vi "Seven Segment Display.vi"(7 "Seven Seg Type (Common Anode)":enum16{"Common Anode", "Common Cathode"}(ring), 8 "Error In":errorcluster, 9 "Character":string="s", 10 "Channels":u8[](array[numeric]), 11 "LINX Resource":T2) -> (0 "Error Out":errorcluster, 2 "Seven Seg Indicator":T1, 3 "LINX Resource":T2)   [LabVIEW 2020, in "LMH-LINX.lvlib"]
doc: "Write a character to a seven segment display using digital output pins. If a multi character string is pass into 'Character' this vi writest he last character. If the selected character cannot be rendered on a seven segment display all segments will turn off."
uses:
  LMH-LINX.lvlib
  Private/Type Defs/LINX Ref.ctl
  Private/Type Defs/Platform.ctl
  Private/Type Defs/Interface.ctl
  Private/Device/Type Defs/LINX Device Config.ctl
  Private/Device/Type Defs/TCP Config.ctl
  Private/Device/Type Defs/Channels.ctl
  Private/Type Defs/Seven Segment Control.ctl
  Peripherals/Digital/Digital Write N Chans.vi
  Private/Local IO/LinxDigitalWrite.vi
  Utilities/Check Channel.vi
  Private/Utilties/Generate Error.vi
  Private/Device/Device.lvlib
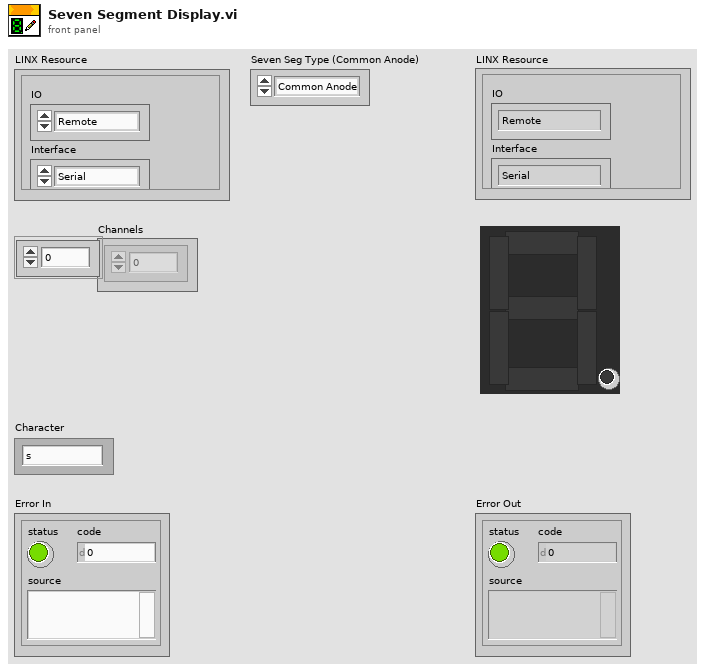
[diagram p1: front panel]
types:
  T1 = typedef "LMH-LINX.lvlib/Seven Segment Control.ctl" = cluster{"Segment 0":bool, "Segment 1":bool, "Segment 2":bool, "Segment 3":bool, "Segment 4":bool, "Segment 5":bool, "Segment 6":bool, "DP":bool}
  T2 = typedef "LMH-LINX.lvlib/LINX Ref.ctl" = cluster{"IO":T3, "Interface":T4, "LINX Device Config":T5}
  T3 = typedef "LMH-LINX.lvlib/Platform.ctl" = enum16{"Remote", "Local"}
  T4 = typedef "LMH-LINX.lvlib/Interface.ctl" = enum16{"Serial", "TCP"}
  T5 = typedef "LMH-LINX.lvlib/Device.lvlib/LINX Device Config.ctl" = cluster{"Interface":T4, "COM Port":refnum<visa-resource-name>, "TCP Configuration":T6, "Device Family":u8, "Device ID":u8, "Device Name":string, "TCP Ref":refnum<k5>, "Channels":T7}
  T6 = typedef "LMH-LINX.lvlib/Device.lvlib/TCP Config.ctl" = cluster{"IP Address":string, "Port":u16}
  T7 = typedef "LMH-LINX.lvlib/Channels.ctl" = cluster{"DI":u8[], "DO":u8[], "AI":u8[], "AO":u8[], "PWM":u8[], "QE":u8[], "UART":u8[], "I2C 2":u8[], "SPI":u8[], "CAN":u8[], "Servo":u8[], "AI Ref (V)":dbl, "AI Resolution (Bits)":u8, "AO Ref (V)":dbl, "AO Resolution (Bits)":u8}
  T8 = cluster{"Seven Segment Display 2[0]":bool, "Seven Segment Display 2[1]":bool, "Seven Segment Display 2[2]":bool, "Seven Segment Display 2[3]":bool, "Seven Segment Display 2[4]":bool, "Seven Segment Display 2[5]":bool, "Seven Segment Display 2[6]":bool, "Seven Segment Display 2[7]":bool}
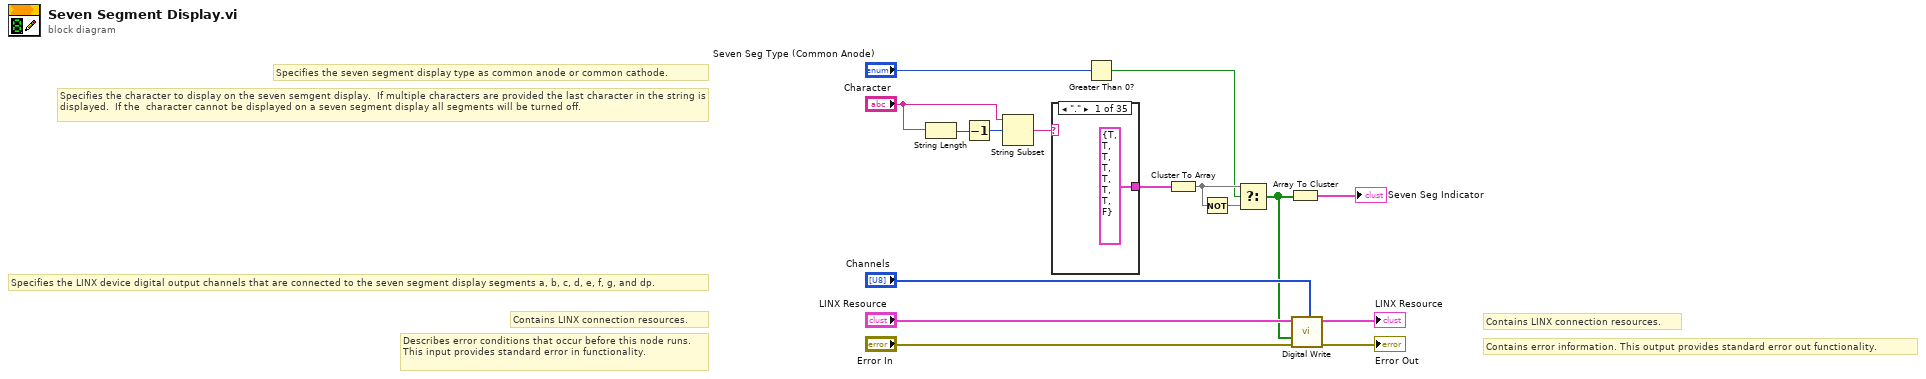
[diagram p0: block diagram]
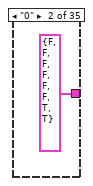
[diagram p2: hidden frame]
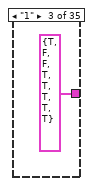
[diagram p3: hidden frame]
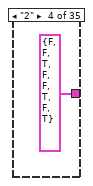
[diagram p4: hidden frame]
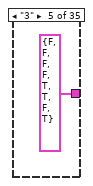
[diagram p5: hidden frame]
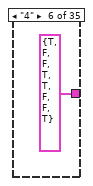
[diagram p6: hidden frame]
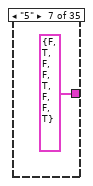
[diagram p7: hidden frame]
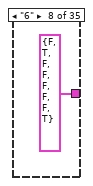
[diagram p8: hidden frame]
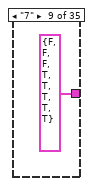
[diagram p9: hidden frame]
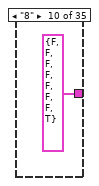
[diagram p10: hidden frame]
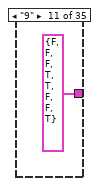
[diagram p11: hidden frame]
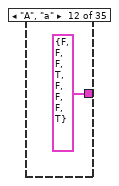
[diagram p12: hidden frame]
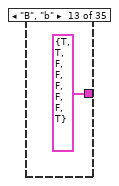
[diagram p13: hidden frame]
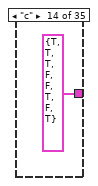
[diagram p14: hidden frame]
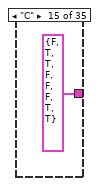
[diagram p15: hidden frame]
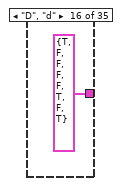
[diagram p16: hidden frame]
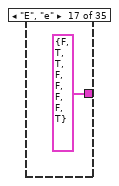
[diagram p17: hidden frame]
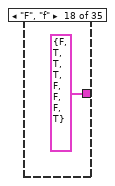
[diagram p18: hidden frame]
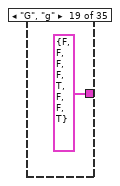
[diagram p19: hidden frame]
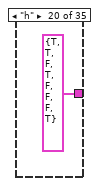
[diagram p20: hidden frame]
diagram:
  # "Specifies the LINX device digital output channels that are connected to the seven segment display segments a, b, c, d, e, f, g, and dp."
  # "Specifies the character to display on the seven semgent display.  If multiple characters are provided the last character in the string is displayed.  If the  character cannot be displayed on a seven segment display all segments will be turned off."
  # "Specifies the seven segment display type as common anode or common cathode."
  # "Contains LINX connection resources."
  # "Contains error information. This output provides standard error out functionality."
  # "Contains LINX connection resources."
  # "Describes error conditions that occur before this node runs. This input provides standard error in functionality."
  n1 = String Length(string="Character") -> (length=w3:i32)
  n2 = Decrement(x=w3) -> (x-1=w2:i32)
  n3 = String Subset(string="Character", offset (0)=w2) -> (substring=w1:string)  [unwired: 1 in]
  n4 = case shown="\".\"" w1 {
    tunnel: [T1 {"Segment 0"=TRUE, "Segment 1"=TRUE, "Segment 2"=TRUE, "Segment 3"=TRUE, "Segment 4"=TRUE, "Segment 5"=TRUE, "Segment 6"=TRUE, "DP"=FALSE} ("Seven Segment Display 2") T1 {"Segment 0"=FALSE, "Segment 1"=FALSE, "Segment 2"=FALSE, "Segment 3"=FALSE, "Segment 4"=FALSE, "Segment 5"=FALSE, "Segment 6"=TRUE, "DP"=TRUE} ("Seven Segment Display 2") T1 {"Segment 0"=TRUE, "Segment 1"=FALSE, "Segment 2"=FALSE, "Segment 3"=TRUE, "Segment 4"=TRUE, "Segment 5"=TRUE, "Segment 6"=TRUE, "DP"=TRUE} ("Seven Segment Display 2") T1 {"Segment 0"=FALSE, "Segment 1"=FALSE, "Segment 2"=TRUE, "Segment 3"=FALSE, "Segment 4"=FALSE, "Segment 5"=TRUE, "Segment 6"=FALSE, "DP"=TRUE} ("Seven Segment Display 2") T1 {"Segment 0"=FALSE, "Segment 1"=FALSE, "Segment 2"=FALSE, "Segment 3"=FALSE, "Segment 4"=TRUE, "Segment 5"=TRUE, "Segment 6"=FALSE, "DP"=TRUE} ("Seven Segment Display 2") T1 {"Segment 0"=TRUE, "Segment 1"=FALSE, "Segment 2"=FALSE, "Segment 3"=TRUE, "Segment 4"=TRUE, "Segment 5"=FALSE, "Segment 6"=FALSE, "DP"=TRUE} ("Seven Segment Display 2") T1 {"Segment 0"=FALSE, "Segment 1"=TRUE, "Segment 2"=FALSE, "Segment 3"=FALSE, "Segment 4"=TRUE, "Segment 5"=FALSE, "Segment 6"=FALSE, "DP"=TRUE} ("Seven Segment Display 2") T1 {"Segment 0"=FALSE, "Segment 1"=TRUE, "Segment 2"=FALSE, "Segment 3"=FALSE, "Segment 4"=FALSE, "Segment 5"=FALSE, "Segment 6"=FALSE, "DP"=TRUE} ("Seven Segment Display 2") T1 {"Segment 0"=FALSE, "Segment 1"=FALSE, "Segment 2"=FALSE, "Segment 3"=TRUE, "Segment 4"=TRUE, "Segment 5"=TRUE, "Segment 6"=TRUE, "DP"=TRUE} ("Seven Segment Display 2") T1 {"Segment 0"=FALSE, "Segment 1"=FALSE, "Segment 2"=FALSE, "Segment 3"=FALSE, "Segment 4"=FALSE, "Segment 5"=FALSE, "Segment 6"=FALSE, "DP"=TRUE} ("Seven Segment Display 2") T1 {"Segment 0"=FALSE, "Segment 1"=FALSE, "Segment 2"=FALSE, "Segment 3"=TRUE, "Segment 4"=TRUE, "Segment 5"=FALSE, "Segment 6"=FALSE, "DP"=TRUE} ("Seven Segment Display 2") T1 {"Segment 0"=FALSE, "Segment 1"=FALSE, "Segment 2"=FALSE, "Segment 3"=TRUE, "Segment 4"=FALSE, "Segment 5"=FALSE, "Segment 6"=FALSE, "DP"=TRUE} ("Seven Segment Display 2") T1 {"Segment 0"=TRUE, "Segment 1"=TRUE, "Segment 2"=FALSE, "Segment 3"=FALSE, "Segment 4"=FALSE, "Segment 5"=FALSE, "Segment 6"=FALSE, "DP"=TRUE} ("Seven Segment Display 2") T1 {"Segment 0"=TRUE, "Segment 1"=TRUE, "Segment 2"=TRUE, "Segment 3"=FALSE, "Segment 4"=FALSE, "Segment 5"=TRUE, "Segment 6"=FALSE, "DP"=TRUE} ("Seven Segment Display 2") T1 {"Segment 0"=FALSE, "Segment 1"=TRUE, "Segment 2"=TRUE, "Segment 3"=FALSE, "Segment 4"=FALSE, "Segment 5"=FALSE, "Segment 6"=TRUE, "DP"=TRUE} ("Seven Segment Display 2") T1 {"Segment 0"=TRUE, "Segment 1"=FALSE, "Segment 2"=FALSE, "Segment 3"=FALSE, "Segment 4"=FALSE, "Segment 5"=TRUE, "Segment 6"=FALSE, "DP"=TRUE} ("Seven Segment Display 2") T1 {"Segment 0"=FALSE, "Segment 1"=TRUE, "Segment 2"=TRUE, "Segment 3"=FALSE, "Segment 4"=FALSE, "Segment 5"=FALSE, "Segment 6"=FALSE, "DP"=TRUE} ("Seven Segment Display 2") T1 {"Segment 0"=FALSE, "Segment 1"=TRUE, "Segment 2"=TRUE, "Segment 3"=TRUE, "Segment 4"=FALSE, "Segment 5"=FALSE, "Segment 6"=FALSE, "DP"=TRUE} ("Seven Segment Display 2") T1 {"Segment 0"=FALSE, "Segment 1"=FALSE, "Segment 2"=FALSE, "Segment 3"=FALSE, "Segment 4"=TRUE, "Segment 5"=FALSE, "Segment 6"=FALSE, "DP"=TRUE} ("Seven Segment Display 2") T1 {"Segment 0"=TRUE, "Segment 1"=TRUE, "Segment 2"=FALSE, "Segment 3"=TRUE, "Segment 4"=FALSE, "Segment 5"=FALSE, "Segment 6"=FALSE, "DP"=TRUE} ("Seven Segment Display 2") T1 {"Segment 0"=TRUE, "Segment 1"=FALSE, "Segment 2"=FALSE, "Segment 3"=TRUE, "Segment 4"=FALSE, "Segment 5"=FALSE, "Segment 6"=FALSE, "DP"=TRUE} ("Seven Segment Display 2") T1 {"Segment 0"=TRUE, "Segment 1"=FALSE, "Segment 2"=FALSE, "Segment 3"=TRUE, "Segment 4"=TRUE, "Segment 5"=TRUE, "Segment 6"=TRUE, "DP"=TRUE} ("Seven Segment Display 2") T1 {"Segment 0"=TRUE, "Segment 1"=FALSE, "Segment 2"=FALSE, "Segment 3"=FALSE, "Segment 4"=FALSE, "Segment 5"=TRUE, "Segment 6"=TRUE, "DP"=TRUE} ("Seven Segment Display 2") T1 {"Segment 0"=TRUE, "Segment 1"=TRUE, "Segment 2"=TRUE, "Segment 3"=FALSE, "Segment 4"=FALSE, "Segment 5"=FALSE, "Segment 6"=TRUE, "DP"=TRUE} ("Seven Segment Display 2") T1 {"Segment 0"=TRUE, "Segment 1"=TRUE, "Segment 2"=FALSE, "Segment 3"=TRUE, "Segment 4"=FALSE, "Segment 5"=TRUE, "Segment 6"=FALSE, "DP"=TRUE} ("Seven Segment Display 2") T1 {"Segment 0"=FALSE, "Segment 1"=FALSE, "Segment 2"=FALSE, "Segment 3"=FALSE, "Segment 4"=FALSE, "Segment 5"=FALSE, "Segment 6"=TRUE, "DP"=TRUE} ("Seven Segment Display 2") T1 {"Segment 0"=TRUE, "Segment 1"=TRUE, "Segment 2"=FALSE, "Segment 3"=FALSE, "Segment 4"=FALSE, "Segment 5"=TRUE, "Segment 6"=FALSE, "DP"=TRUE} ("Seven Segment Display 2") T1 {"Segment 0"=FALSE, "Segment 1"=FALSE, "Segment 2"=TRUE, "Segment 3"=TRUE, "Segment 4"=FALSE, "Segment 5"=FALSE, "Segment 6"=FALSE, "DP"=TRUE} ("Seven Segment Display 2") T1 {"Segment 0"=FALSE, "Segment 1"=FALSE, "Segment 2"=FALSE, "Segment 3"=TRUE, "Segment 4"=TRUE, "Segment 5"=FALSE, "Segment 6"=FALSE, "DP"=TRUE} ("Seven Segment Display 2") T1 {"Segment 0"=TRUE, "Segment 1"=TRUE, "Segment 2"=TRUE, "Segment 3"=TRUE, "Segment 4"=FALSE, "Segment 5"=TRUE, "Segment 6"=FALSE, "DP"=TRUE} ("Seven Segment Display 2") T1 {"Segment 0"=FALSE, "Segment 1"=TRUE, "Segment 2"=FALSE, "Segment 3"=FALSE, "Segment 4"=TRUE, "Segment 5"=FALSE, "Segment 6"=FALSE, "DP"=TRUE} ("Seven Segment Display 2") T1 {"Segment 0"=TRUE, "Segment 1"=TRUE, "Segment 2"=FALSE, "Segment 3"=FALSE, "Segment 4"=FALSE, "Segment 5"=TRUE, "Segment 6"=TRUE, "DP"=TRUE} ("Seven Segment Display 2") T1 {"Segment 0"=TRUE, "Segment 1"=FALSE, "Segment 2"=FALSE, "Segment 3"=FALSE, "Segment 4"=FALSE, "Segment 5"=FALSE, "Segment 6"=TRUE, "DP"=TRUE} ("Seven Segment Display 2") T1 {"Segment 0"=TRUE, "Segment 1"=FALSE, "Segment 2"=FALSE, "Segment 3"=FALSE, "Segment 4"=TRUE, "Segment 5"=FALSE, "Segment 6"=FALSE, "DP"=TRUE} ("Seven Segment Display 2") T1 {"Segment 0"=FALSE, "Segment 1"=FALSE, "Segment 2"=FALSE, "Segment 3"=FALSE, "Segment 4"=FALSE, "Segment 5"=FALSE, "Segment 6"=FALSE, "DP"=FALSE} ("Seven Segment Display 2")] -> w16
    frame "." {
    }
    frame "0" {
    }
    frame "1" {
    }
    frame "2" {
    }
    frame "3" {
    }
    frame "4" {
    }
    frame "5" {
    }
    frame "6" {
    }
    frame "7" {
    }
    frame "8" {
    }
    frame "9" {
    }
    frame "A", "a" {
    }
    frame "B", "b" {
    }
    frame "c" {
    }
    frame "C" {
    }
    frame "D", "d" {
    }
    frame "E", "e" {
    }
    frame "F", "f" {
    }
    frame "G", "g" {
    }
    frame "h" {
    }
    frame "H" {
    }
    frame "I", "i" {
    }
    frame "J", "j" {
    }
    frame "L", "l" {
    }
    frame "N", "n" {
    }
    frame "O" {
    }
    frame "o" {
    }
    frame "P", "p" {
    }
    frame "Q", "q" {
    }
    frame "R", "r" {
    }
    frame "S", "s" {
    }
    frame "u" {
    }
    frame "U" {
    }
    frame "Y", "y" {
    }
    frame " ", Default {
    }
  }
  n5 = Greater Than 0?(x="Seven Seg Type (Common Anode)") -> (x > 0?=w12:bool)
  n6 = Cluster To Array(cluster=w16) -> (array=w15:bool[])
  n7 = Not(x=w15) -> (.not. x?=w14:bool[])
  n8 = Select(t=w15, s=w12, f=w14) -> (s? t:f=w7:bool[])
  n9 = Array To Cluster(array=w7) -> (cluster=→"Seven Seg Indicator":T8)
  n10 = call-poly "Digital Write.vi"("Error In"="Error In", "Values"=w7, "DO Channels"="Channels", "LINX Resource"="LINX Resource") -> ("Error Out"=→"Error Out":errorcluster, "LINX Resource"=→"LINX Resource":T2)  [unwired: 6 in]
